vi "XML Script - Shift Register.vi"(2 "out":i32=-1, 4 "location":T1, 6 "name":string, 8 "offset":i32=1, 9 "prefix (name)":string, 10 "in":i32=-1) -> (5 "name (wire source)":string, 7 "XML Script Command - Tunnel":string)   [LabVIEW 2017]
uses:
  <vilib>/_script/XML Scripting/Structure Location.ctl
  <vilib>/_script/XML Scripting/XML Script Tag.ctl
  <vilib>/_script/XML Scripting/XML Script Attribute.ctl
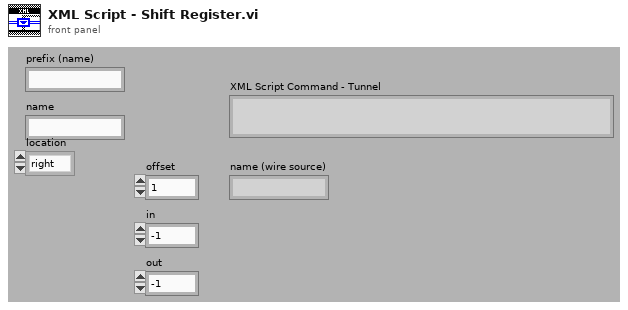
[diagram p1: front panel]
types:
  T1 = typedef "Structure Location.ctl" = enum16{"right", "left", "top", "bottom"}
  T2 = typedef "XML Script Attribute.ctl" = enum16{"name", "style", "path", "position", "in", "out", "width", "height", "index", "value", "default", "location", "offset", "typeindex", "size", "source", "destination", "indicator", "type", "controlname", "label", "conpaneidx", "mode", "description", "hasCondTerm", "linkIdentity", "caseselectortype", "concatInputs", "inName", "instantiationpath", "loopCondition", "IndexMode", "formulaInputs", "formulaOutputs", "msnFuncName", "msnIsDynamic", "msnIsODEUserFunction", "ignoreSearchDialog"}
  T3 = typedef "XML Script Tag.ctl" = enum16{"Script", "Function", "SubVI", "GrowableFunction", "Structure", "MultiframeStructure", "Frame", "Tunnel", "ShiftRegister", "Constant", "Control", "Terminal", "Wire", "StaticVIReference", "ControlTerminal", "CompoundArithmetic", "FlatSequence", "FlatSequenceFrame", "MathScriptCallByRef", "BuildArray", "GenericSubVI", "MathScriptNode"}
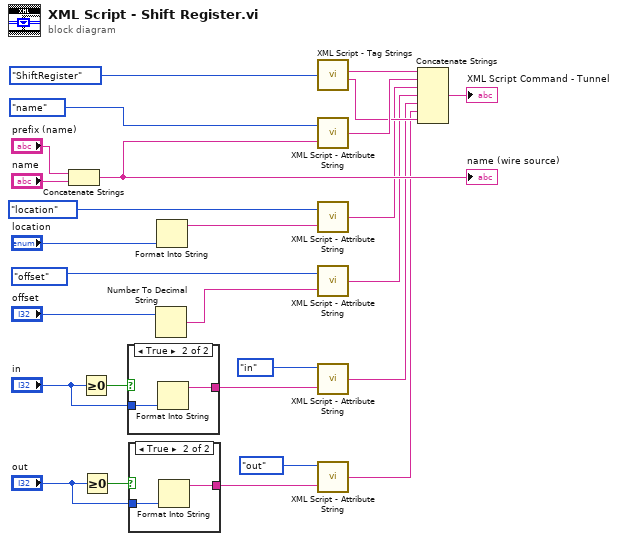
[diagram p0: block diagram]
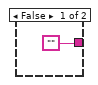
[diagram p2: hidden frame]
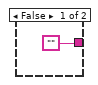
[diagram p3: hidden frame]
diagram:
  n1 = Concatenate Strings("prefix (name)", "name") -> (w17:string)
  "name (wire source)" <- w17
  n2 = Greater Or Equal To 0?(x="in") -> (x >= 0?=w7:bool)
  n3 = Greater Or Equal To 0?(x="out") -> (x >= 0?=w11:bool)
  n4 = case shown="True" w7 {
    tunnel: "in" -> [_ w30]
    tunnel: ["" w29] -> w9
    frame False {
    }
    frame True {
      n5 = Format Into String(w30) -> (resulting string=w29:string)  [unwired: 3 in, 1 out]
    }
  }
  n6 = case shown="True" w11 {
    tunnel: "out" -> [_ w33]
    tunnel: ["" w32] -> w13
    frame False {
    }
    frame True {
      n7 = Format Into String(w33) -> (resulting string=w32:string)  [unwired: 3 in, 1 out]
    }
  }
  n8 = Number To Decimal String(number="offset") -> (decimal integer string=w14:string)  [unwired: 1 in]
  n9 = Format Into String("location") -> (resulting string=w20:string)  [unwired: 3 in, 1 out]
  n10 = call <vilib>:"XML Script - Tag Strings.vi"("XML Script Tag"=XML_Script_Tag."ShiftRegister") -> ("XML String - Begin Tag"=w24:string, "XML String - End Tag"=w5:string)  [unwired: 2 in]
  n11 = call <vilib>:"XML Script - Attribute String.vi"("Attribute String"=w17, "XML Script Attribute"=XML_Script_Attribute."name") -> ("XML Script - Attribute String"=w22:string)
  n12 = call <vilib>:"XML Script - Attribute String.vi"("Attribute String"=w20, "XML Script Attribute"=XML_Script_Attribute."location") -> ("XML Script - Attribute String"=w1:string)
  n13 = call <vilib>:"XML Script - Attribute String.vi"("Attribute String"=w14, "XML Script Attribute"=XML_Script_Attribute."offset") -> ("XML Script - Attribute String"=w2:string)
  n14 = call <vilib>:"XML Script - Attribute String.vi"("Attribute String"=w9, "XML Script Attribute"=XML_Script_Attribute."in") -> ("XML Script - Attribute String"=w4:string)
  n15 = call <vilib>:"XML Script - Attribute String.vi"("Attribute String"=w13, "XML Script Attribute"=XML_Script_Attribute."out") -> ("XML Script - Attribute String"=w3:string)
  n16 = Concatenate Strings(w24, w22, w1, w2, w4, w3, w5) -> (→"XML Script Command - Tunnel":string)
